vi "Close.vi"(8 "error in (no error)":errorcluster, 11 "SigGen_ESG in":refnum<class "SigGen_ESG.lvclass">) -> (0 "error out":errorcluster)   [LabVIEW 2014, in "SigGen_ESG.lvclass"]
uses:
  SigGen_ESG.lvclass
  SigGen_ESG.lvclass/SigGen_ESG.ctl
  <instrlib>/Agilent ESG Series/Agilent ESG Series.lvlib
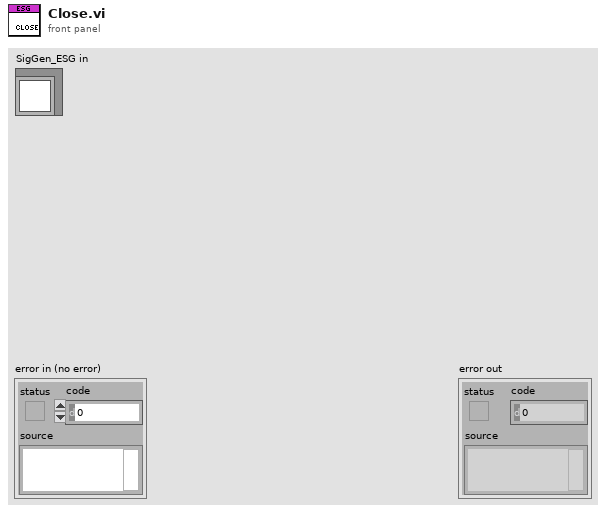
[diagram p1: front panel]
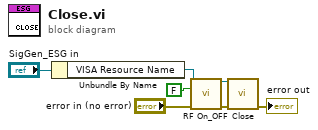
[diagram p0: block diagram]
diagram:
  n1 = Unbundle By Name("SigGen_ESG in") -> ("VISA Resource Name"=w5:refnum<visa-resource-name>)
  n2 = call <instrlib>:"RF On_OFF.vi"("VISA Resource Name"=w5, "Status (T:ON)"=FALSE, "error in (no error)"="error in (no error)") -> ("VISA Resource Name Out"=w2:refnum<visa-resource-name>, "error out"=w1:errorcluster)  [unwired: 11 in]
  n3 = call <instrlib>:"Close.vi"("VISA Resource Name"=w2, "error in (no error)"=w1) -> ("error out"=→"error out":errorcluster)  [unwired: 13 in]
